vi "Basic Usage of Loki Logger.vi"() -> ()   [LabVIEW 2017]
uses:
  HSE-Logger/Handler/LokiHandler/LokiHandler.lvclass
  C:/Projects/HSE Logger/Source/HSE-Logger/Handler/Handler.lvclass
  HSE-Logger/hse-logger.lvlib
panel:
  in  "error in":errorcluster
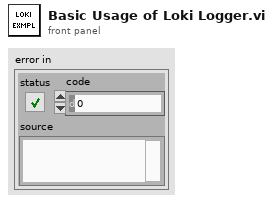
[diagram p1: front panel]
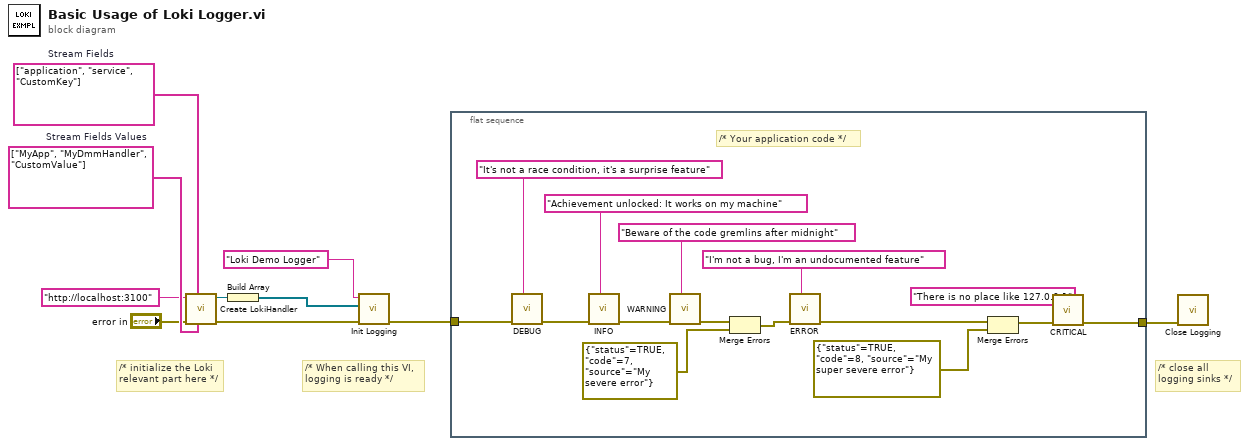
[diagram p0: block diagram]
diagram:
  w7 = string[] ["MyApp", "MyDmmHandler", "CustomValue"]  # Stream Fields Values
  w6 = string[] ["application", "service", "CustomKey"]  # Stream Fields
  # "/* close all \nlogging sinks */"
  # "/* When calling this VI,\nlogging is ready */"
  # "/* initialize the Loki\nrelevant part here */"
  n1 = call "Create LokiHandler.vi"("Stream Fields Values"=w7, "Stream Fields"=w6, "error in"="error in", "Loki URL and Port"="http://localhost:3100") -> ("error out"=w3:errorcluster, "LokiHandler out"=w10:refnum<class "LokiHandler.lvclass">)  [unwired: 6 in]
  n2 = Build Array(w10) -> (w9:refnum<class "LokiHandler.lvclass">[])
  n3 = call "Init Logging.vi"("error in"=w3, "Handlers"=w9, "Name"="Loki Demo Logger") -> ("error out"=w2:errorcluster)  [unwired: 8 in]
  n4 = flat-sequence {
    tunnel: w2 -> [w25]
    tunnel: [w11] -> w1
    frame #0 {
      # "/* Your application code */"
      n5 = call "DEBUG.vi"("Message"="It's not a race condition, it's a surprise feature", "error in"=w25) -> ("error out"=w23:errorcluster)  [unwired: 9 in]
      n6 = call "INFO.vi"("Message"="Achievement unlocked: It works on my machine", "error in"=w23) -> ("error out"=w21:errorcluster)  [unwired: 9 in]
      n7 = call "WARNING.vi"("Message"="Beware of the code gremlins after midnight", "error in"=w21) -> ("error out"=w19:errorcluster)  [unwired: 9 in]
      n8 = Merge Errors(w19, errorcluster {"status"=TRUE, "code"=7, "source"="My severe error"} ("error in")) -> (w18:errorcluster)
      n9 = call "ERROR.vi"("Message"="I'm not a bug, I'm an undocumented feature", "error in"=w18) -> ("error out"=w14:errorcluster)  [unwired: 9 in]
      n10 = Merge Errors(w14, errorcluster {"status"=TRUE, "code"=8, "source"="My super severe error"} ("error in")) -> (w13:errorcluster)
      n11 = call "CRITICAL.vi"("Message"="There is no place like 127.0.0.1", "error in"=w13) -> ("error out"=w11:errorcluster)  [unwired: 9 in]
    }
  }
  n12 = call "Close Logging.vi"("error in"=w1) -> ()  [unwired: 10 in, 1 out]
